vi "ValidateXML.vi"(8 "error in":errorcluster, 11 "Value in":string) -> (0 "error out":errorcluster, 3 "Value out":string)   [LabVIEW 2021, in "ProligentXMLGenerator.lvlib" / "CustomElement.lvclass"]
uses:
  CustomElement.lvclass
  CustomElement.lvclass/CustomElement.ctl
  <vilib>/xml/NI_XML.lvlib
  <resource>/objmgr/DOMUserDefRef.rc
  <vilib>/xml/Close Reference(Node).vi
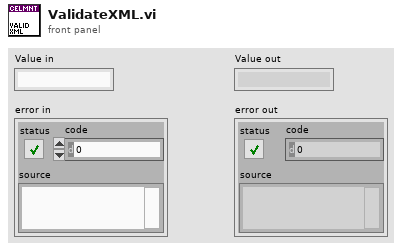
[diagram p1: front panel]
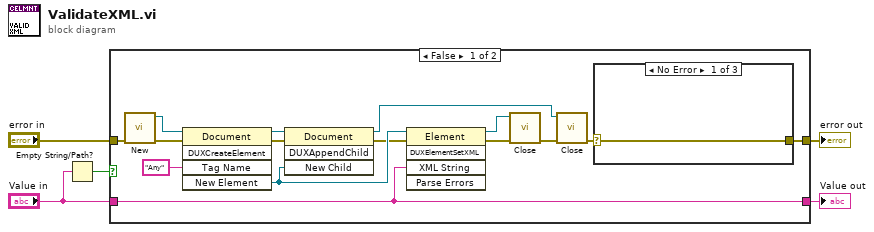
[diagram p0: block diagram]
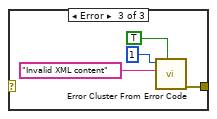
[diagram p3: hidden frame]
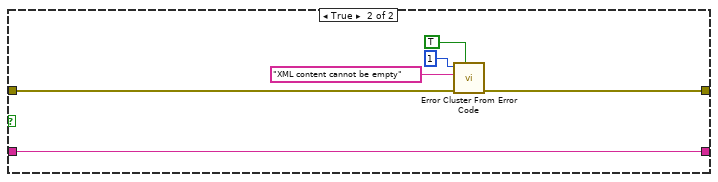
[diagram p4: hidden frame]
diagram:
  n1 = Empty String/Path?(string/path="Value in") -> (empty?=w1:bool)
  n2 = case shown="False" w1 {
    tunnel: [w10 w27] -> w5
    tunnel: "error in" -> [w9 w28]
    tunnel: "Value in" -> [w8 w32]
    tunnel: [w8 w32] -> w2
    frame False {
      n3 = call <vilib>:"New.vi"("error in (no error)"=w9) -> ("error out"=w20:errorcluster, "DOM document out"=w17:refnum<k20>)  [unwired: 7 in]
      n4 = invoke class="Document" method="DUXCreateElement"(reference=w17, error in=w20, "Tag Name"="Any") -> (reference out=w15:refnum<k20>, error out=w19:errorcluster, "New Element"=w13:refnum<k20>)  [unwired: 2 in, 2 out]
      n5 = invoke class="Document" method="DUXAppendChild"(reference=w15, error in=w19, "New Child"=w13) -> (reference out=w14:refnum<k20>, error out=w12:errorcluster)  [unwired: 1 in, 2 out]
      n6 = invoke class="Element" method="DUXElementSetXML"(reference=w13, error in=w12, "XML String"=w8) -> (reference out=w7:refnum<k20>, error out=w6:errorcluster)  [unwired: 2 in, 3 out]
      n7 = call-poly <vilib>:"Close.vi"("error in (no error)"=w6, "node"=w7) -> ("error out"=w16:errorcluster)  [unwired: 7 in]
      n8 = call-poly <vilib>:"Close.vi"("error in (no error)"=w16, "node"=w14) -> ("error out"=w11:errorcluster)  [unwired: 7 in]
      n9 = case shown="No Error" w11 {
        selector: w11 -> [w21 w22 _]
        tunnel: [w21 w22 w26] -> w10
        frame No Error {
        }
        frame Default {
        }
        frame Error {
          n10 = call <vilib>:"Error Cluster From Error Code.vi"("show call chain? (False)"=TRUE, "error message (\"\")"="Invalid XML content", "error code (0)"=1) -> ("error out"=w26:errorcluster)  [unwired: 6 in]
        }
      }
    }
    frame True {
      n11 = call <vilib>:"Error Cluster From Error Code.vi"("show call chain? (False)"=TRUE, "error in (no error)"=w28, "error message (\"\")"="XML content cannot be empty", "error code (0)"=1) -> ("error out"=w27:errorcluster)  [unwired: 5 in]
    }
  }
  "error out" <- w5
  "Value out" <- w2
